vi "driveLogicTester.vi"() -> ()   [LabVIEW 2017]
uses:
  Drive Logic/driveLogicStates.ctl
panel:
  in  "approachedElement":bool
  in  "toGuidedDrive":bool
  in  "toApproachingElement":bool
  in  "toTurnAngle":bool
  in  "toFreestyle":bool
  in  "toDriveDistance":bool
  in  "toDoNothing":bool
  out "Current state":T1
  in  "stop":bool
  # "If the boolean is flicked up, and the state allows the transition,\nthe current state will transition to that state."
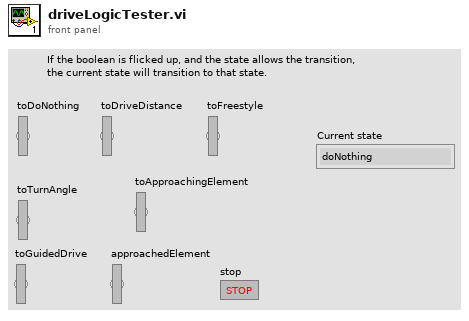
[diagram p1: front panel]
types:
  T1 = typedef "driveLogicStates.ctl" = enum16{"doNothing", "driveDistance", "turnAngle", "freestyle", "guidedDrive", "approachingElement"}
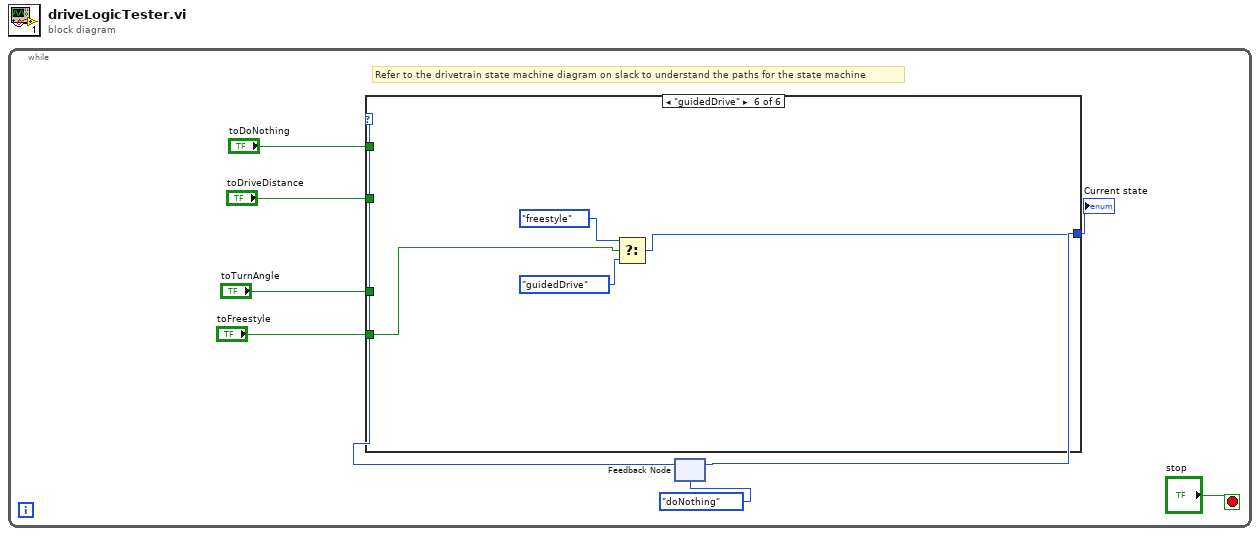
[diagram p0: block diagram]
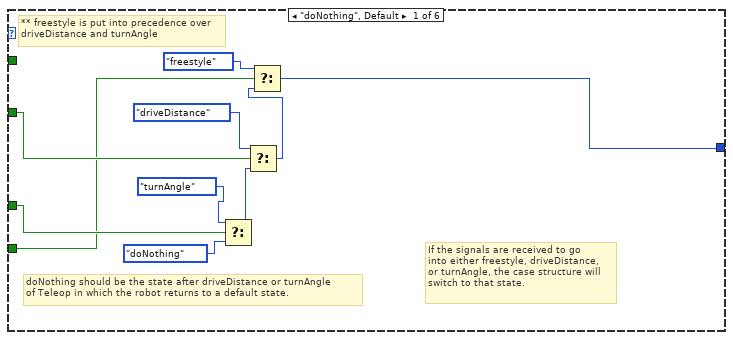
[diagram p2: hidden frame]
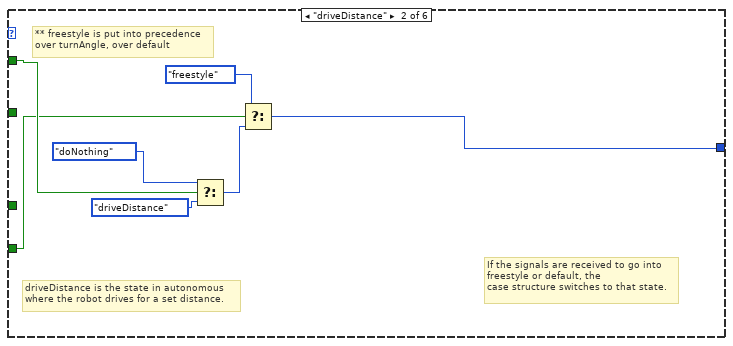
[diagram p3: hidden frame]
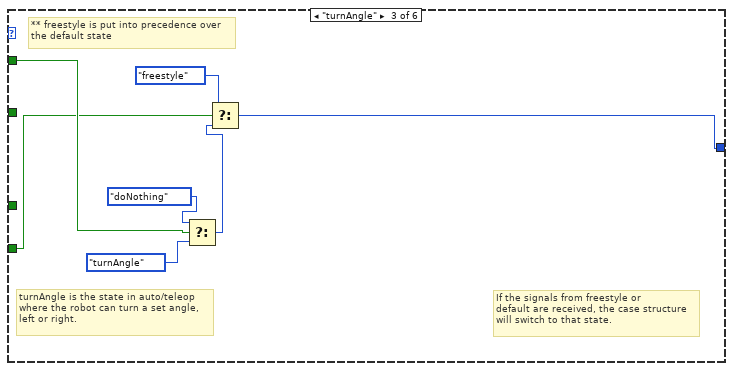
[diagram p4: hidden frame]
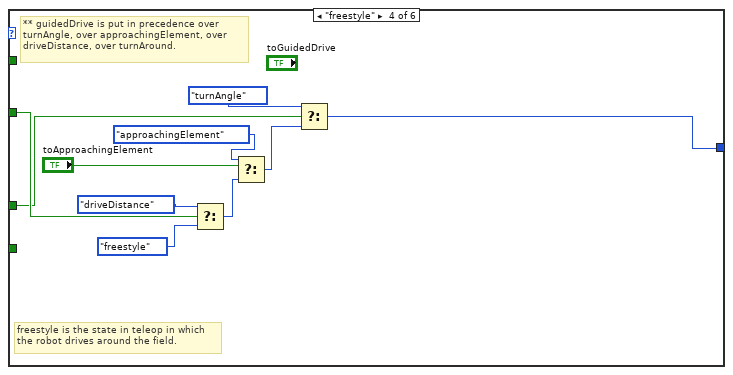
[diagram p5: hidden frame]
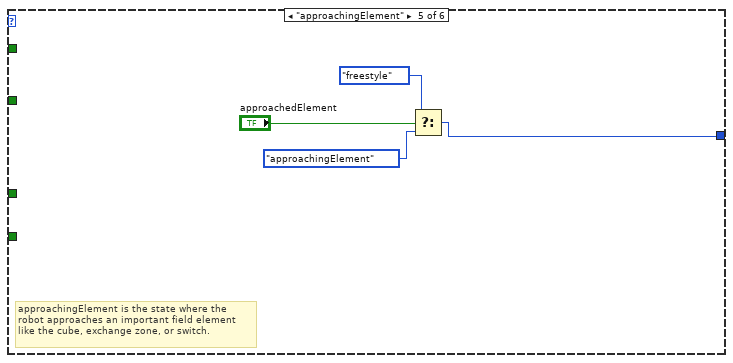
[diagram p6: hidden frame]
diagram:
  n1 = while {
    stop <- "stop" stop-if-true
    # "Refer to the drivetrain state machine diagram on slack to understand the paths for the state machine"
    n2 = feedback #1(driveLogicStates."doNothing") -> (w8:T1)
    n3 = case shown="\"guidedDrive\"" w8 {
      tunnel: [w16 w23 w31 w37 w44 w47] -> w6
      tunnel: "toDoNothing" -> [_ w20 w27 _ _ _]
      tunnel: "toDriveDistance" -> [w10 _ _ w35 _ _]
      tunnel: "toTurnAngle" -> [w11 _ _ w34 _ _]
      tunnel: "toFreestyle" -> [w9 w19 w26 _ _ w50]
      frame "doNothing", Default {
        # "** freestyle is put into precedence over\ndriveDistance and turnAngle"
        # "If the signals are received to go\ninto either freestyle, driveDistance,\nor turnAngle, the case structure will\nswitch to that state."
        # "doNothing should be the state after driveDistance or turnAngle \nof Teleop in which the robot returns to a default state."
        n4 = Select(t=driveLogicStates."turnAngle", s=w11, f=driveLogicStates."doNothing") -> (s? t:f=w18:T1)
        n5 = Select(t=driveLogicStates."driveDistance", s=w10, f=w18) -> (s? t:f=w17:T1)
        n6 = Select(t=driveLogicStates."freestyle", s=w9, f=w17) -> (s? t:f=w16:T1)
      }
      frame "driveDistance" {
        # "If the signals are received to go into\nfreestyle or default, the\ncase structure switches to that state."
        # "** freestyle is put into precedence\nover turnAngle, over default"
        # "driveDistance is the state in autonomous\nwhere the robot drives for a set distance."
        n7 = Select(t=driveLogicStates."doNothing", s=w20, f=driveLogicStates."driveDistance") -> (s? t:f=w21:T1)
        n8 = Select(t=driveLogicStates."freestyle", s=w19, f=w21) -> (s? t:f=w23:T1)
      }
      frame "turnAngle" {
        # "If the signals from freestyle or\ndefault are received, the case structure\nwill switch to that state."
        # "turnAngle is the state in auto/teleop\nwhere the robot can turn a set angle,\nleft or right."
        # "** freestyle is put into precedence over\nthe default state"
        n9 = Select(t=driveLogicStates."doNothing", s=w27, f=driveLogicStates."turnAngle") -> (s? t:f=w29:T1)
        n10 = Select(t=driveLogicStates."freestyle", s=w26, f=w29) -> (s? t:f=w31:T1)
      }
      frame "freestyle" {
        # "freestyle is the state in teleop in which \nthe robot drives around the field."
        # "** guidedDrive is put in precedence over\nturnAngle, over approachingElement, over\ndriveDistance, over turnAround."
        n11 = Select(t=driveLogicStates."driveDistance", s=w35, f=driveLogicStates."freestyle") -> (s? t:f=w40:T1)
        n12 = Select(t=driveLogicStates."approachingElement", s="toApproachingElement", f=w40) -> (s? t:f=w41:T1)
        n13 = Select(t=driveLogicStates."turnAngle", s=w34, f=w41) -> (s? t:f=w37:T1)
      }
      frame "approachingElement" {
        # "approachingElement is the state where the \nrobot approaches an important field element\nlike the cube, exchange zone, or switch."
        n14 = Select(t=driveLogicStates."freestyle", s="approachedElement", f=driveLogicStates."approachingElement") -> (s? t:f=w44:T1)
      }
      frame "guidedDrive" {
        n15 = Select(t=driveLogicStates."freestyle", s=w50, f=driveLogicStates."guidedDrive") -> (s? t:f=w47:T1)
      }
    }
    "Current state" <- w6
    n16 = feedback-in #1(w6) -> ()
  }
